vi "Go_to_State3.vi"(8 "error in (no error)":errorcluster, 11 "State3 in":refnum<class "State3.lvclass">) -> (0 "error out":errorcluster, 3 "State out":refnum<class "State Actor.lvclass">)   [LabVIEW 2025, in "Demo_States.lvlib" / "State3.lvclass"]
uses:
  State3.lvclass
  State3.lvclass/State3.ctl
  Demo_States/Demo_States.lvclass
  <vilib>/ni/Actors/State Actor/State Actor/State Actor.lvclass
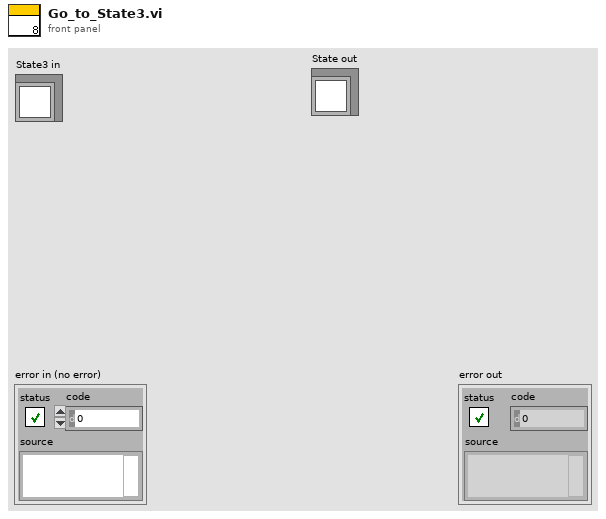
[diagram p1: front panel]
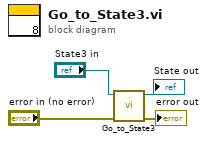
[diagram p0: block diagram]
diagram:
  n1 = call-parent "Go_to_State3.vi"("error in (no error)"="error in (no error)", "Demo_States in"="State3 in") -> ("error out"=→"error out":errorcluster, "State out"=→"State out":refnum<class "State Actor.lvclass">)  [unwired: 8 in]
